vi "XYZ Get Position.vi"(8 "error in (no error)":errorcluster, 10 "Pos In in":dbl[](array[numeric]), 11 "LSID":i32) -> (0 "error out":errorcluster, 2 "Pos In out":dbl[](array[numeric]))   [LabVIEW 2014]
uses:
  <userlib>/Tango_DLL/Tango_DLL.lvlib
panel:
  # "LICENSED MATERIALS – PROPERTY OF IBM\nCopyright IBM Corp. 2016,\nALL RIGHTS RESERVED"
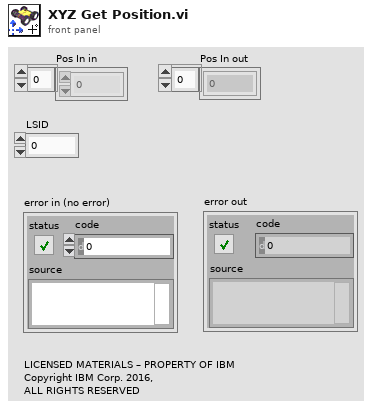
[diagram p1: front panel]
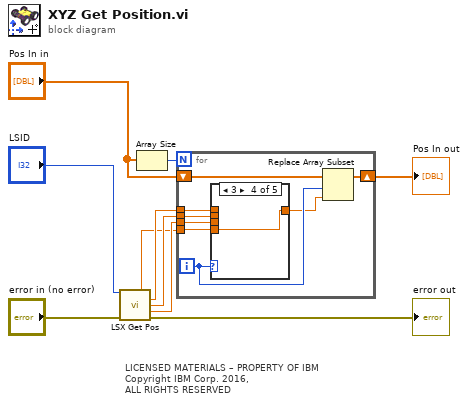
[diagram p0: block diagram]
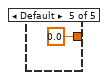
[diagram p5: hidden frame]
diagram:
  # "LICENSED MATERIALS – PROPERTY OF IBM\nCopyright IBM Corp. 2016,\nALL RIGHTS RESERVED"
  n1 = call <userlib>:"LSX Get Pos.vi"("lLSID"="LSID", "error in (no error)"="error in (no error)") -> ("pdA out"=w3:dbl, "pdX out"=w6:dbl, "pdY out"=w5:dbl, "pdZ out"=w4:dbl, "error out"=→"error out":errorcluster)  [unwired: 8 in, 1 out]
  n2 = Array Size(array="Pos In in") -> (size(s)=w7:i32)
  n3 = for {
    N: w7 -> [_]
    tunnel: w6 -> [w17]
    tunnel: w5 -> [w16]
    tunnel: w4 -> [w15]
    tunnel: w3 -> [w14]
    shift-right: [w11] -> w10
    shift-left: "Pos In in" -> [w18]
    i -> [w13]
    n4 = case shown="3" w13 {
      tunnel: w17 -> [w19 _ _ _ _]
      tunnel: w16 -> [_ w20 _ _ _]
      tunnel: w15 -> [_ _ w21 _ _]
      tunnel: w14 -> [_ _ _ w22 _]
      tunnel: [w19 w20 w21 w22 0.0 ("pdA out")] -> w12
      frame 0 {
      }
      frame 1 {
      }
      frame 2 {
      }
      frame 3 {
      }
      frame Default {
      }
    }
    n5 = Replace Array Subset(array=w18, new element=w12, index=w13) -> (w11:dbl[])
  }
  "Pos In out" <- w10
